vi "dynamicData.vi"() -> ()   [LabVIEW 2014]
uses:
  <vilib>/express/express signal manip/GetorSetDDTAttributes/Shared VIs/TimeType.ctl
  <vilib>/express/express signal manip/GetorSetDDTAttributes/Shared VIs/XDimension.ctl
  <vilib>/express/express shared/transition.llb/Dynamic To Waveform Array.vi
  <vilib>/express/express signal manip/GetorSetDDTAttributes/Shared VIs/XDimension conversion.vi
  <vilib>/express/express signal manip/GetorSetDDTAttributes/Get DDT Attributes/Get DDT Properties.xnode
  <vilib>/express/express signal manip/GetorSetDDTAttributes/Shared VIs/GetSetShared.lvlib
panel:
  out "Unit":string
  out "X Dimension":T1
  out "Start Timestamp":timestamp
  out "Timestamp":timestamp
  out "Time Mode":T2
  out "Signal Name":string
  in  "Frequency":dbl(knob)=10.1 scale=0.0..10.0
  in  "Terminate While Loop":bool
  out "Waveform Chart":dynamicdata(graph)
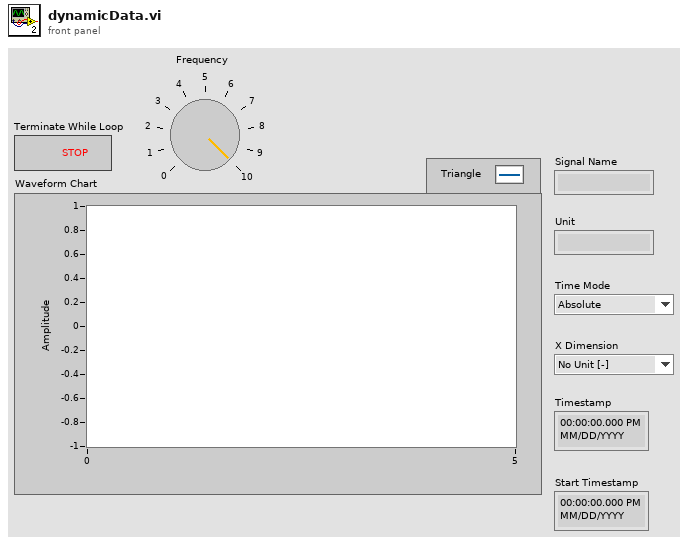
[diagram p1: front panel]
types:
  T1 = typedef "GetSetShared.lvlib/XDimension.ctl" = enum16{"No Unit [-]", "Time [sec]", "Frequency [Hz]"}
  T2 = typedef "GetSetShared.lvlib/TimeType.ctl" = enum16{"Absolute", "Relative"}
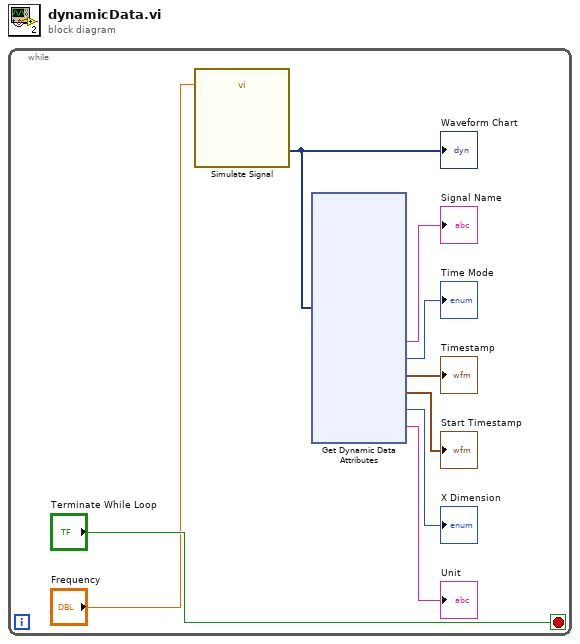
[diagram p0: block diagram]
diagram:
  n1 = while {
    stop <- "Terminate While Loop" stop-if-true
    n2 = call "Simulate Signal"("Frequency"="Frequency") -> ("Triangle"=w7:dynamicdata)  [unwired: 13 in, 1 out]
    "Waveform Chart" <- w7
    n3 = xnode "Get Dynamic Data Attributes"("Signals In"=w7) -> ("Signal Name"=→"Signal Name":string, "Time Mode"=→"Time Mode":T2, "Timestamp"=→"Timestamp":timestamp, "Start Timestamp"=→"Start Timestamp":timestamp, "X Dimension"=→"X Dimension":T1, "Unit"=→"Unit":string)  [unwired: 2 in, 2 out]
  }
